vi "测试.vi"(1 "error in (no error)":cluster{"状态":bool, "代码":i32, "源":string} caption="错误输入（无错误）", 2 "状态通知器":refnum<notifier>) -> (0 "error out":cluster{"状态":bool, "代码":i32, "源":string} caption="错误输出")   [LabVIEW 2014]
uses:
  <vilib>/picture/3D Picture Control/Object/Add Object (reference).vi
  <vilib>/picture/3D Picture Control/NI_3D Picture Control.lvlib
panel:
  in  "Color 2":T1={"Red"=1.0, "Green"=0.0, "Blue"=0.0, "Alpha"=1.0} caption="颜色"
  in  "缩放":dbl(knob)=2.2771854734286614 scale=0.0..10.0
  out "三维图片":refnum<vi>(3d-picture)
  out "动力":dbl(slide) scale=10.0..13.0
  out "back_camera_ip":string
  in  "后摄像头":refnum<k7>(container)
  in  "主摄像头":refnum<k7>(container)
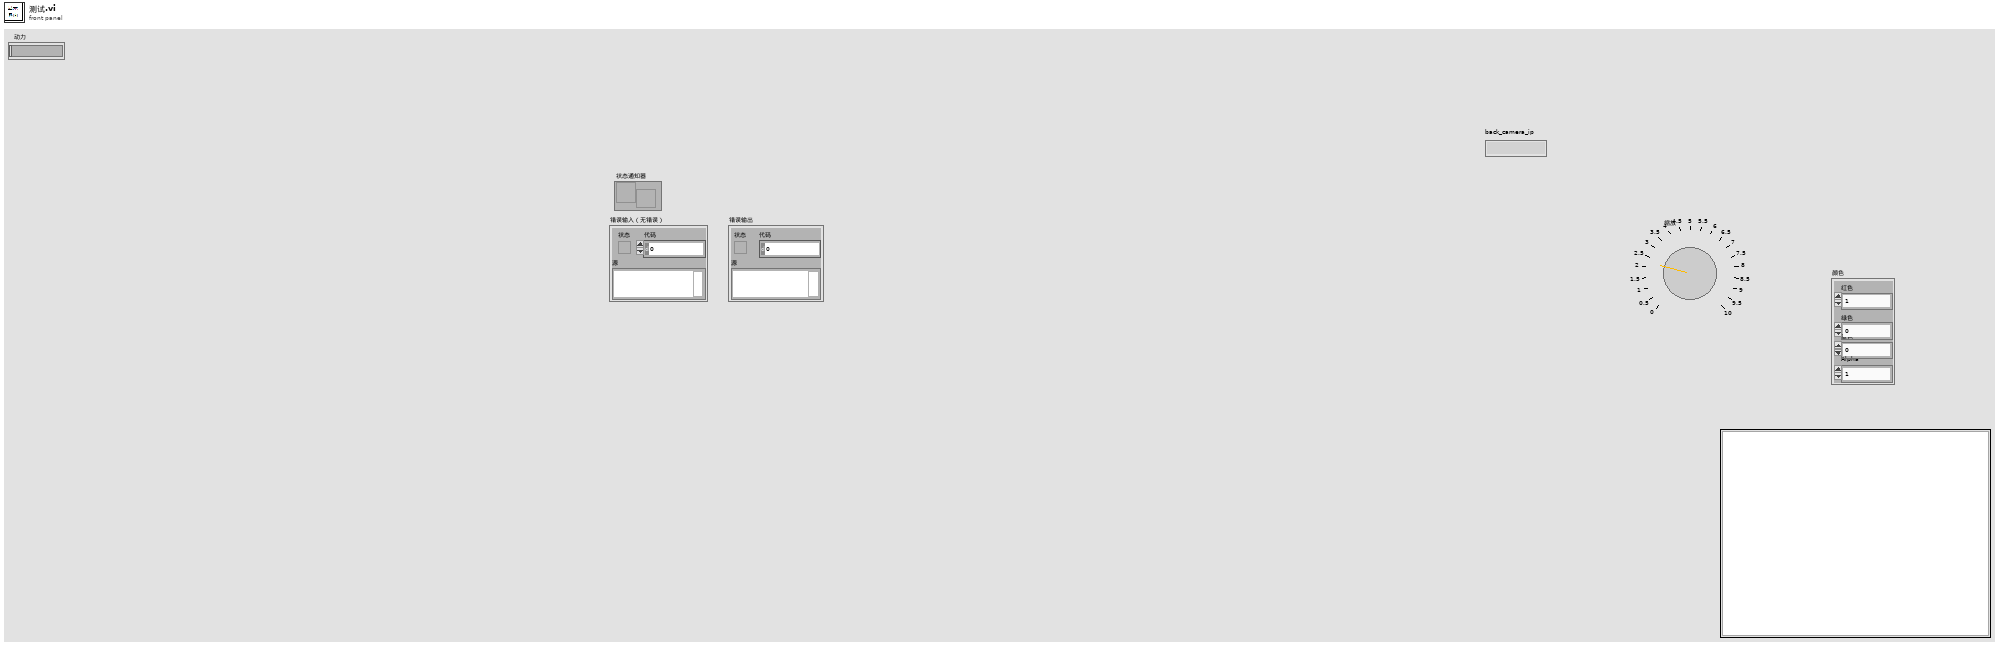
[diagram p1: front panel]
types:
  T1 = cluster{"Red":sgl, "Green":sgl, "Blue":sgl, "Alpha":sgl}
  T2 = cluster{"car_ip":u32, "car_port":i32, "wire_ip":u32, "wire_port":u32, "local_port":u32, "main_camera_ip":string, "back_camera_ip":string}
  T3 = enum32{"Bad", "Idle", "Run top level", "Running"}
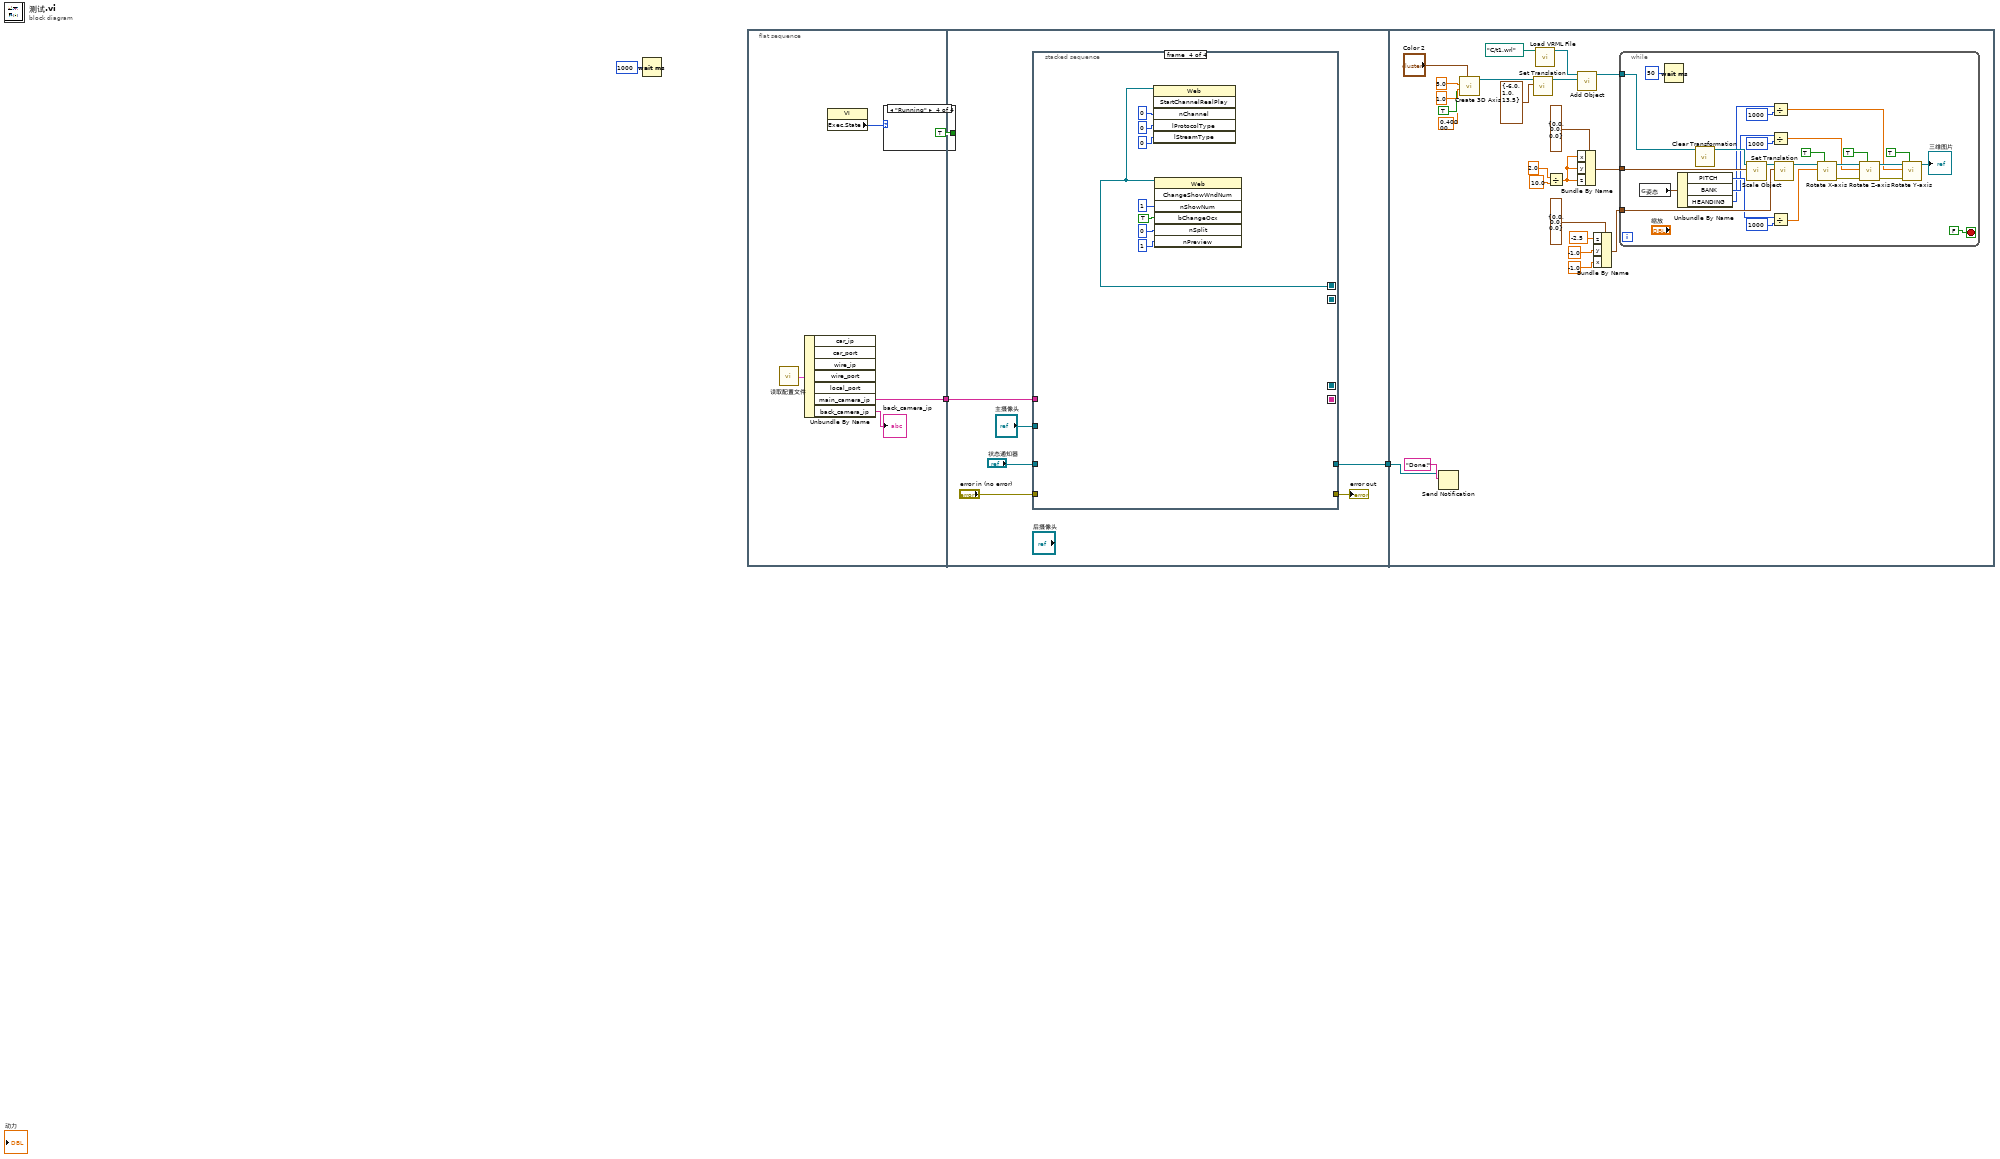
[diagram p0: block diagram]
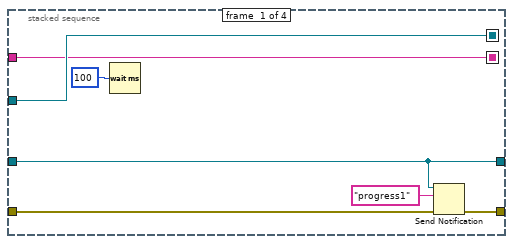
[diagram p2: hidden frame]
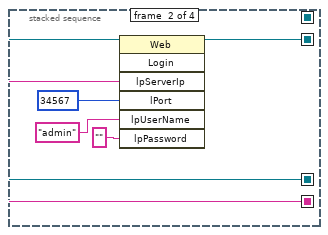
[diagram p3: hidden frame]
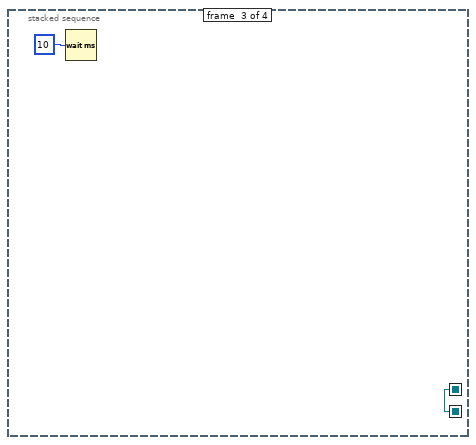
[diagram p4: hidden frame]
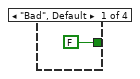
[diagram p5: hidden frame]
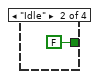
[diagram p6: hidden frame]
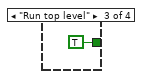
[diagram p7: hidden frame]
diagram:
  n1 = Wait (ms)(milliseconds to wait=u32 1000 ("等待时间（毫秒）")) -> ()  [unwired: 1 out]
  n2 = flat-sequence {
    tunnel: [w6] -> w4
    tunnel: w4 -> [w9]
    tunnel: [w8] -> w3
    tunnel: w3 -> [w37]
    frame #0 {
      n3 = call "读取配置文件.vi"() -> ("簇"=w7:T2)  [unwired: 1 in]
      n4 = Unbundle By Name(w7) -> ("main_camera_ip"=w6:string, "back_camera_ip"=→"back_camera_ip":string)  [unwired: 5 out]
    }
    frame #1 {
      n5 = stacked-sequence {
        seq-local: [w20 _ _ _] -> [_ w25 _ _]
        seq-local: [w19 _ _ _] -> [_ w24 _ _]
        seq-local: [_ w26 _ _] -> [_ _ w28 _]
        seq-local: [_ _ w28 _] -> [_ _ _ w36]
        tunnel: "主摄像头" -> [w20 _ _ _]
        tunnel: w9 -> [w19 _ _ _]
        tunnel: "状态通知器" -> [w14 _ _ _]
        tunnel: "error in (no error)" -> [w17 _ _ _]
        tunnel: [w15 _ _ _] -> w10
        tunnel: [w14 _ _ _] -> w8
        frame #0 {
          n6 = Wait (ms)(milliseconds to wait=u32 100 ("等待时间（毫秒）")) -> ()  [unwired: 1 out]
          n7 = Send Notification(notification="progress1", notifier=w14, error in (no error)=w17) -> (error out=w15:errorcluster)  [unwired: 1 out]
        }
        frame #1 {
          n8 = invoke class="Web" method="Login"(reference=w25, "lpServerIp"=w24, "lPort"=34567, "lpUserName"="admin", "lpPassword"="") -> (reference out=w26:refnum<k7>)  [unwired: 2 in, 6 out]
        }
        frame #2 {
          n9 = Wait (ms)(milliseconds to wait=u32 10 ("等待时间（毫秒）")) -> ()  [unwired: 1 out]
        }
        frame #3 {
          n10 = invoke class="Web" method="StartChannelRealPlay"(reference=w36, "nChannel"=0, "lProtocolType"=0, "lStreamType"=0) -> ()  [unwired: 2 in, 6 out]
          n11 = invoke class="Web" method="ChangeShowWndNum"(reference=w36, "nShowNum"=1, "bChangeOcx"=TRUE, "nSplit"=0, "nPreview"=1) -> ()  [unwired: 2 in, 7 out]
        }
      }
      "error out" <- w10
    }
    frame #2 {
      n12 = Send Notification(notification="Done!", notifier=w37) -> ()  [unwired: 1 in, 2 out]
      n13 = call <vilib>:"Create 3D Axis.vi"("Character Size"=sgl 0.4, "Axis label?"=TRUE, "Color"="Color 2", "Radius"=sgl 1.0, "Length"=sgl 5.0) -> ("New Object Refnum"=w51:refnum<vi>)  [unwired: 5 in, 1 out]
      n14 = call <vilib>:"Set Translation.vi"("Translation"=cluster{"X":sgl, "Y":sgl, "Z":sgl} {"X"=-6.0, "Y"=1.0, "Z"=13.5}, "Scene Object"=w51) -> ("Translated Object"=w50:refnum<vi>)  [unwired: 8 in, 1 out]
      n15 = call <vilib>:"Load VRML File.vi"("Path"=path "C:/t1.wrl" ("路径")) -> ("Scene:Read Scene File"=w53:refnum<vi>)  [unwired: 9 in, 1 out]
      n16 = Divide(x=2.0, y=10.0) -> (x/y=w43:dbl)
      n17 = call-poly <vilib>:"Add Object.vi"("New Object In"=w50, "Scene Object In"=w53) -> ("Scene Object Out"=w55:refnum<vi>)  [unwired: 7 in, 2 out]
      n18 = Bundle By Name(cluster=cluster{"x":dbl, "y":dbl, "z":dbl} {"x"=0.0, "y"=0.0, "z"=0.0}, "x"=w43, "y"=w43, "z"=w43) -> (w41:cluster{"x":dbl, "y":dbl, "z":dbl})
      n19 = Bundle By Name(cluster=cluster{"x":dbl, "y":dbl, "z":dbl} {"x"=0.0, "y"=0.0, "z"=0.0}, "z"=-2.5, "y"=-1.0, "x"=-1.0) -> (w48:cluster{"x":dbl, "y":dbl, "z":dbl})
      n20 = while {
        tunnel: w55 -> [w68]
        tunnel: w48 -> [w67]
        tunnel: w41 -> [w66]
        stop <- FALSE stop-if-true
        n21 = global read "全局变量.vi" "姿态"() -> (w63:cluster{"PITCH":i32, "BANK":i32, "HEANDING":i32})
        n22 = Wait (ms)(milliseconds to wait=u32 50 ("等待时间（毫秒）")) -> ()  [unwired: 1 out]
        n23 = Unbundle By Name(w63) -> ("PITCH"=w62:i32, "BANK"=w61:i32, "HEANDING"=w60:i32)
        n24 = call <vilib>:"Clear Transformation.vi"("Object Refnum In"=w68) -> ("Object Refnum Out"=w69:refnum<vi>)  [unwired: 9 in, 1 out]
        n25 = call <vilib>:"Scale Object.vi"("Scale"=w66, "Scene.Object In"=w69) -> ("Scene.Object Out"=w84:refnum<vi>)  [unwired: 8 in, 1 out]
        n26 = Divide(x=w60, y=1000) -> (x/y=w71:dbl)
        n27 = Divide(x=w61, y=1000) -> (x/y=w73:dbl)
        n28 = Divide(x=w62, y=1000) -> (x/y=w72:dbl)
        n29 = call <vilib>:"Set Translation.vi"("Translation"=w67, "Scene Object"=w84) -> ("Translated Object"=w81:refnum<vi>)  [unwired: 8 in, 1 out]
        n30 = call <vilib>:"Rotate X-axis.vi"("Relative?"=TRUE, "angle"=w72, "Scene Object In"=w81) -> ("error out"=w80:errorcluster, "Scene Object Out"=w79:refnum<vi>)  [unwired: 7 in]
        n31 = call <vilib>:"Rotate Z-axis.vi"("Relative?"=TRUE, "error in (no error)"=w80, "angle"=w73, "Scene Object In"=w79) -> ("error out"=w76:errorcluster, "Scene Object Out"=w75:refnum<vi>)  [unwired: 6 in]
        n32 = call <vilib>:"Rotate Y-axis.vi"("Relative?"=TRUE, "error in (no error)"=w76, "angle"=w71, "Scene Object In"=w75) -> ("Scene Object Out"=→"三维图片":refnum<vi>)  [unwired: 6 in, 1 out]
      }
    }
  }
  n33 = property class="VI"() -> ("Exec.State"=w1:T3)  [unwired: 2 in, 2 out]
  n34 = case shown="\"Running\"" w1 {
    tunnel: [FALSE FALSE TRUE TRUE] -> _
    frame "Bad", Default {
    }
    frame "Idle" {
    }
    frame "Run top level" {
    }
    frame "Running" {
    }
  }
